vi "Restart.SaveSettings.vi"(8 "error in":errorcluster, 10 "Restart Settings":T1={"LogFile"=path "", "Log Settings"=[], "StimulusProfile"=path "", "StopIteration"=0, "StopStep"=0, "Log Channels"=enum."Aliases", "Base File Name"="Log", "Enable Logging"=TRUE, "Profile"="", "StopDuration"=0.0}, 11 "datalog path (use dialog)":path) -> (0 "error out":errorcluster, 3 "path":path)   [LabVIEW 2013, in "Simple Sequence Tools - Execution.lvlib"]
uses:
  Simple Sequence Tools - Execution.lvlib
  Types/Restart.Settings
  <vilib>/NI Veristand/Execution/DataLogging/TDMS Channel Group.ctl
  <vilib>/NI Veristand/Execution/DataLogging/TDMS Property.ctl
  <vilib>/NI Veristand/Execution/DataLogging/TDMS Channel.ctl
  <vilib>/NI Veristand/Execution/DataLogging/Time Channel Options.ctl
  Types/Log.SelectedChannels.ctl
  Shared/SubVIs/Main.Constants.vi
  <vilib>/NI/GXML/GXML.lvlib
  Shared/Simple Sequence Tools - Shared.lvlib
  <vilib>/NI Veristand/Execution/DataLogging/NI_VS Data Logging API.lvlib
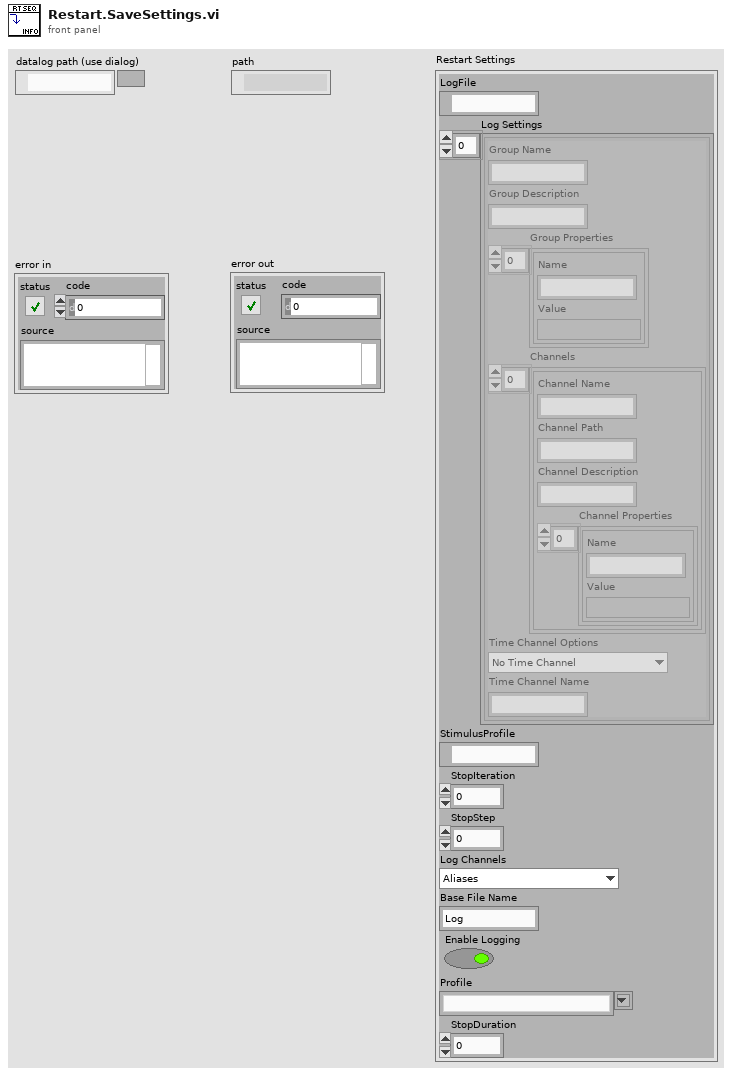
[diagram p1: front panel]
types:
  T1 = typedef "Simple Sequence Tools - Execution.lvlib/Restart.Settings" = cluster{"LogFile":path, "Log Settings":T2[], "StimulusProfile":path, "StopIteration":u32, "StopStep":u32, "Log Channels":T6, "Base File Name":string, "Enable Logging":bool, "Profile":string, "StopDuration":dbl}
  T2 = typedef "NI_VS Data Logging API.lvlib/TDMS Channel Group.ctl" = cluster{"Group Name":string, "Group Description":string, "Group Properties":T3[], "Channels":T4[], "Time Channel Options":T5, "Time Channel Name":string}
  T3 = typedef "NI_VS Data Logging API.lvlib/TDMS Property.ctl" = cluster{"Name":string, "Value":variant}
  T4 = typedef "NI_VS Data Logging API.lvlib/TDMS Channel.ctl" = cluster{"Channel Name":string, "Channel Path":string, "Channel Description":string, "Channel Properties":T3[]}
  T5 = typedef "NI_VS Data Logging API.lvlib/Time Channel Options.ctl" = enum16{"No Time Channel", "Absolute Time", "System Time", "System Time - Microseconds", "Absolute Time as Double"}
  T6 = typedef "Simple Sequence Tools - Execution.lvlib/Log.SelectedChannels.ctl" = enum16{"Channels (No System Channel)", "Aliases", "All"}
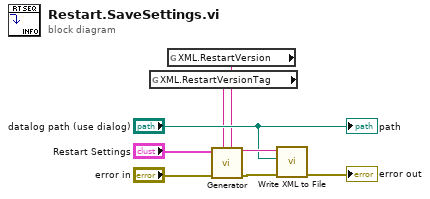
[diagram p0: block diagram]
diagram:
  n1 = global read "Main.Constants.vi" "XML.RestartVersionTag"() -> (w2:string)
  n2 = global read "Main.Constants.vi" "XML.RestartVersion"() -> (w1:string)
  n3 = call <vilib>:"Generator.vi"("Version String"=w1, "Version Tag Name"=w2, "error in"="error in", "Variant"="Restart Settings") -> ("error out"=w7:errorcluster, "XML String Out"=w8:string)  [unwired: 6 in]
  n4 = call <vilib>:"Write XML to File.vi"("error in"=w7, "XML File Path"="datalog path (use dialog)", "XML Input"=w8) -> ("error out"=→"error out":errorcluster)  [unwired: 8 in]
  "path" <- "datalog path (use dialog)"
